vi "Current step.vi"(8 "error in (no error)":errorcluster, 11 "Stepping Function in":refnum<class "Stepping Function.lvclass">) -> (0 "error out":errorcluster, 2 "Step value":refnum<class "Mag Lab Result.lvclass">, 3 "Stepping Function out":refnum<class "Stepping Function.lvclass">)   [LabVIEW 2015, in "Stepping Function.lvclass"]
uses:
  Stepping Function.lvclass
  Mag Lab Result/Mag Lab Result.lvclass
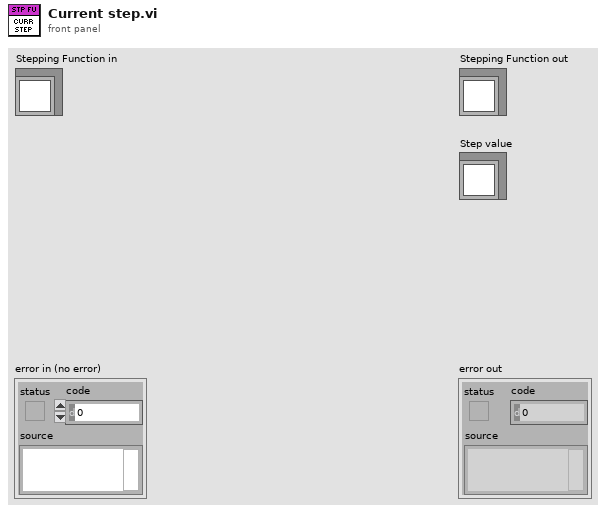
[diagram p1: front panel]
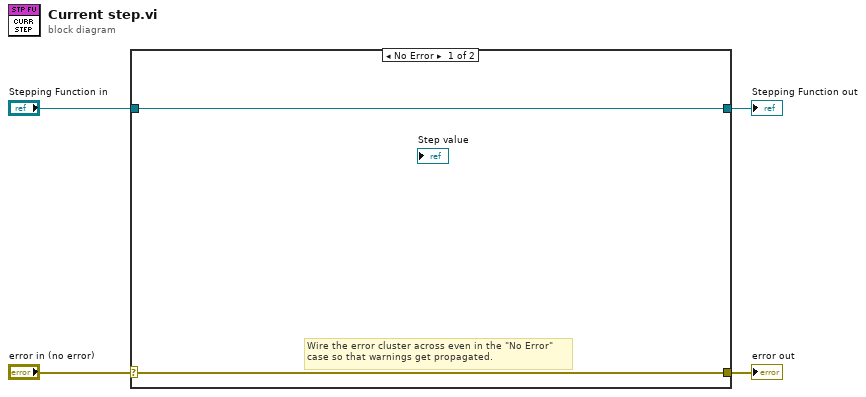
[diagram p0: block diagram]
diagram:
  n1 = case shown="No Error" "error in (no error)" {
    selector: "error in (no error)" -> [w5 w8]
    tunnel: [w5 w8] -> w3
    tunnel: [w6 w7] -> w1
    tunnel: "Stepping Function in" -> [w6 w7]
    frame No Error {
      # "Wire the error cluster across even in the \"No Error\"\ncase so that warnings get propagated."
    }
    frame Error {
    }
  }
  "error out" <- w3
  "Stepping Function out" <- w1
